vi "writeToXMLElevation.vi"(8 "error in (no error)":errorcluster, 10 "Class Label":string="Elevation") -> (0 "error out":errorcluster, 2 "XML out":string="<>\n  <degreesAlt>90</degreesAlt>\n  <minutesArc>0</minutesArc>\n  <secondsArc>0</secondsArc>\n</>")   [LabVIEW 2012]
uses:
  <userlib>/Common/UnitsAndXML/FlattenItemWithUnitToXML/FlattenPlaneAngleToXML/PlaneAngleUnit.ctl
  <userlib>/Common/UnitsAndXML/UnitsAndXML.lvlib
  <userlib>/Common/XML/XMLAttributeGenerator/XMLAttributeGenerator.lvclass
panel:
  in  "secondsArc":dbl[unit]=0.0002617993877991494
  in  "minutesArc":dbl[unit]=0.00930842267730309
  in  "degreesAlt":dbl[unit]=0.7330382858376184
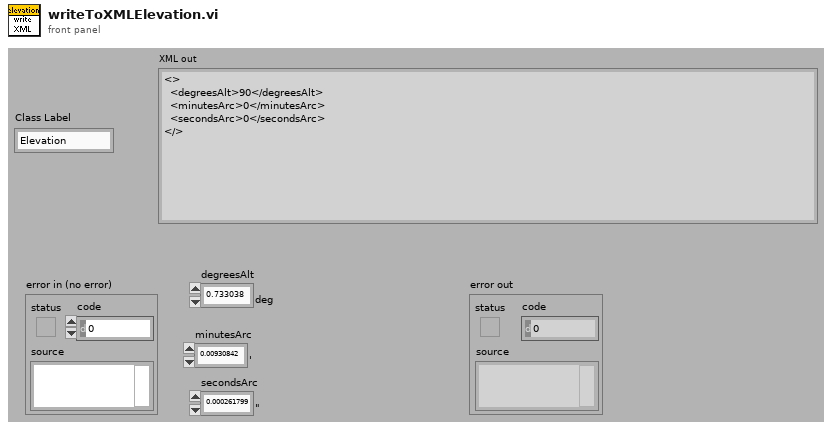
[diagram p1: front panel]
types:
  T1 = typedef "UnitsAndXML.lvlib/PlaneAngleUnit.ctl" = enum16{"rad", "deg", "'", "\""}
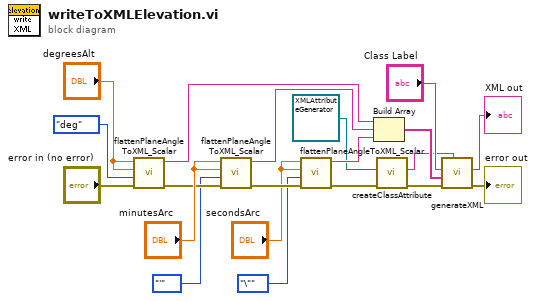
[diagram p0: block diagram]
diagram:
  n1 = call <userlib>:"flattenPlaneAngleToXML_Scalar.vi"("error in (no error)"="error in (no error)", "planeAngleUnitInXML"=PlaneAngleUnit."deg", "planeAngleAgain"="degreesAlt", "planeAngle"="degreesAlt") -> ("error out"=w17:errorcluster, "xmlString"=w12:string)  [unwired: 6 in]
  n2 = call <userlib>:"flattenPlaneAngleToXML_Scalar.vi"("error in (no error)"=w17, "planeAngleUnitInXML"=PlaneAngleUnit."'", "planeAngleAgain"="minutesArc", "planeAngle"="minutesArc") -> ("error out"=w16:errorcluster, "xmlString"=w11:string)  [unwired: 6 in]
  n3 = call <userlib>:"flattenPlaneAngleToXML_Scalar.vi"("error in (no error)"=w16, "planeAngleUnitInXML"=PlaneAngleUnit."\"", "planeAngleAgain"="secondsArc", "planeAngle"="secondsArc") -> ("error out"=w5:errorcluster, "xmlString"=w6:string)  [unwired: 6 in]
  n4 = Build Array(w12, w11, w6) -> (w10:string[])
  n5 = call <userlib>:"createClassAttribute.vi"("error in (no error)"=w5, "LVClass In"=refnum<class "XMLAttributeGenerator.lvclass"> refnum ("WriteAttribute.lvclass")) -> ("error out"=w3:errorcluster, "AttributeString"=w1:string)  [unwired: 7 in, 1 out]
  n6 = call <userlib>:"generateXML.vi"("attributeString"=w1, "error in"=w3, "childrenXML"=w10, "elementName"="Class Label") -> ("error out"=→"error out":errorcluster, "XML out"=→"XML out":string)  [unwired: 5 in, 1 out]
